vi "cmc-mechanical encoder-out.vi"() -> ()   [LabVIEW 2010]
panel:
  in  "stop":bool
  out "Position #":u32
  out "Encoder Bit Values":bool[](array[boolean])
  # "Bit 0"
  # "Bit 1"
  # "Bit 2"
  # "Bit 3"
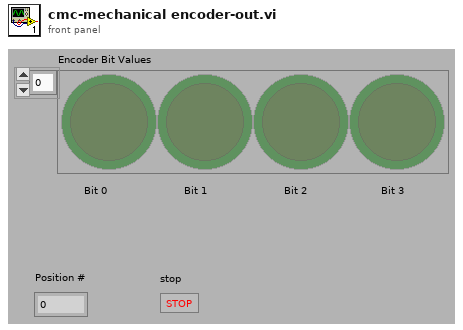
[diagram p1: front panel]
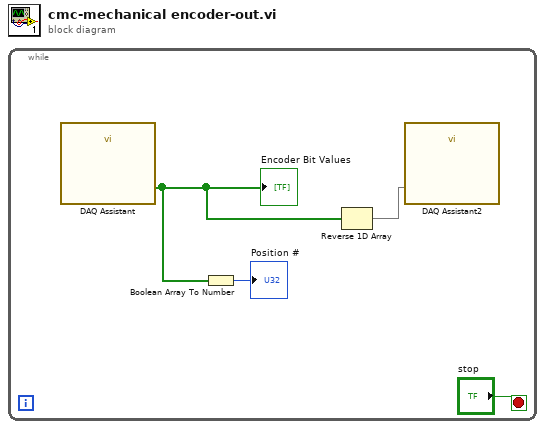
[diagram p0: block diagram]
diagram:
  n1 = while {
    stop <- "stop" stop-if-true
    n2 = call "DAQ Assistant"() -> ("data"=w2:bool[])  [unwired: 17 in, 2 out]
    "Encoder Bit Values" <- w2
    n3 = Boolean Array To Number(Boolean array=w2) -> (number=→"Position #":u32)
    n4 = Reverse 1D Array(array=w2) -> (reversed array=w1:bool[])
    n5 = call "DAQ Assistant2"("data"=w1) -> ()  [unwired: 17 in, 2 out]
  }
